vi "test Duplicate.vi"(8 "error in (no error)":errorcluster, 11 "TestCase In":refnum<class "Data Manipulation Tests.lvclass">) -> (0 "error out":errorcluster, 3 "TestCase Out":refnum<class "Data Manipulation Tests.lvclass">)   [LabVIEW 2017, in "Pointer Tests.lvlib" / "Data Manipulation Tests.lvclass"]
uses:
  Data Manipulation Tests.lvclass
  Source/Classes/Pointer/Public/New/New (4B).vi
  Source/Classes/Pointer/Public/Write/Write (1D I32).vi
  <vilib>/addons/_JKI Toolkits/VI Tester/TestCase.llb/TestCase.lvclass
  Source/Classes/Pointer/Pointer.lvclass
  C:/Program Files (x86)/National Instruments/LabVIEW 2017/vi.lib/addons/_JKI Toolkits/VI Tester/TestCase.llb/TestCase.lvclass
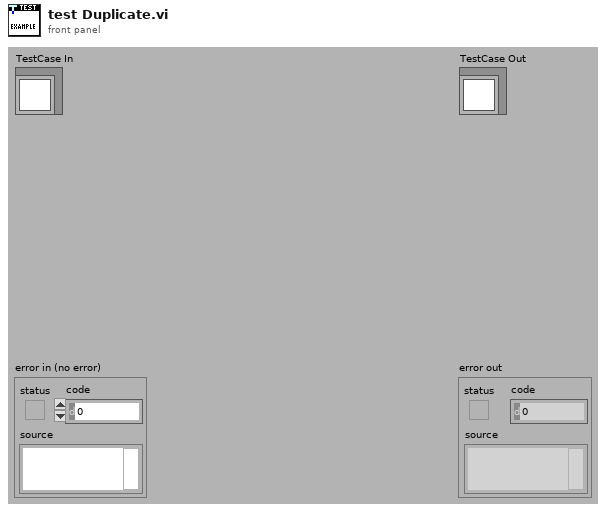
[diagram p1: front panel]
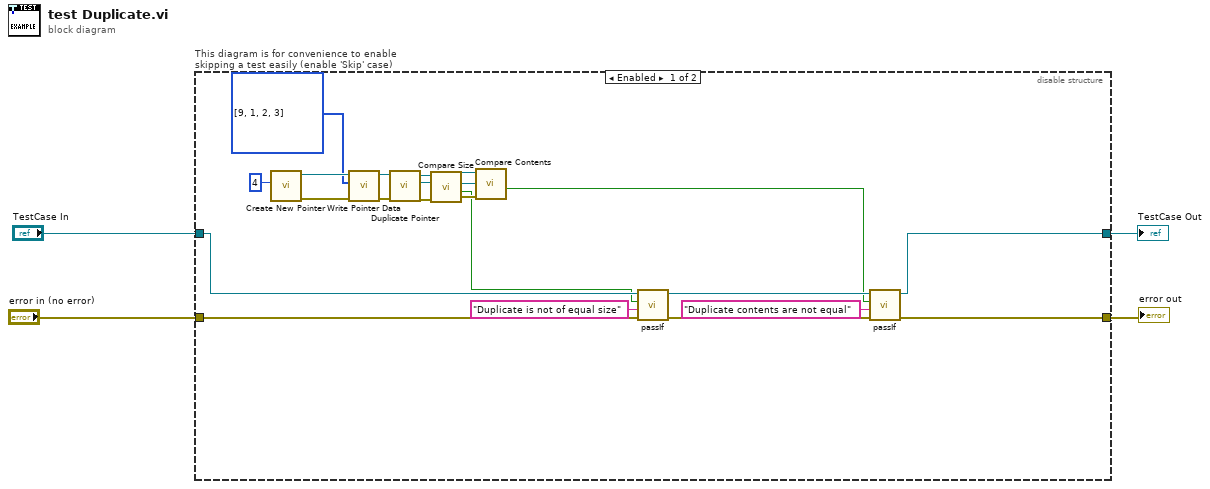
[diagram p0: block diagram]
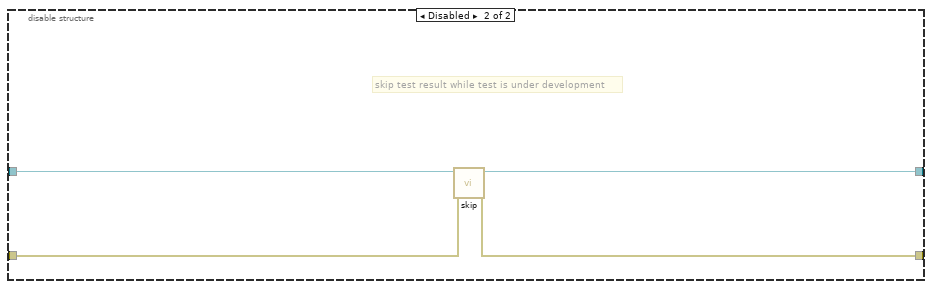
[diagram p2: hidden frame]
diagram:
  n1 = disable-structure "This diagram is for convenience to enable skipping a test easily (enable 'Skip' case)" shown="Enabled" {
    disable-tunnel: "TestCase In" -> [w23 w30]
    disable-tunnel: [w20 w28] -> w1
    disable-tunnel: [w22 w29] -> w3
    disable-tunnel: "error in (no error)" -> [w26 w27]
    frame Enabled {
      n2 = call-poly "Create New Pointer.vi"("count (1)"=u64 4) -> ("error out"=w8:errorcluster, "Pointer"=w25:refnum<class "Pointer.lvclass">)  [unwired: 9 in]
      n3 = call-poly "Write Pointer Data.vi"("error in (no error)"=w8, "buffer in"=i32[] [9, 1, 2, 3] ("count (1)"), "Pointer in"=w25) -> ("error out"=w7:errorcluster, "Pointer out"=w9:refnum<class "Pointer.lvclass">)  [unwired: 5 in, 2 out]
      n4 = call "Duplicate Pointer.vi"("error in (no error)"=w7, "Pointer in"=w9) -> ("error out"=w16:errorcluster, "new duplicate Pointer"=w13:refnum<class "Pointer.lvclass">, "Pointer out"=w17:refnum<class "Pointer.lvclass">)  [unwired: 7 in]
      n5 = call "Compare Size.vi"("error in (no error)"=w16, "Pointer b in"=w13, "Pointer a in"=w17) -> ("error out"=w14:errorcluster, "equal size?"=w11:bool, "Pointer b out"=w12:refnum<class "Pointer.lvclass">, "Pointer a out"=w15:refnum<class "Pointer.lvclass">)  [unwired: 5 in]
      n6 = call "Compare Contents.vi"("error in (no error)"=w14, "Pointer b in"=w12, "Pointer a in"=w15) -> ("equal contents?"=w10:bool)  [unwired: 5 in, 3 out]
      n7 = call-dynamic "passIf.vi"("error in (no error)"=w26, "message (\"\")"="Duplicate is not of equal size" ("message (\"\")"), "pass"=w11, "TestCase in"=w23) -> ("error out"=w24:errorcluster, "TestCase out"=w21:refnum<class "Data Manipulation Tests.lvclass">)  [unwired: 6 in]
      n8 = call-dynamic "passIf.vi"("error in (no error)"=w24, "message (\"\")"="Duplicate contents are not equal" ("message (\"\")"), "pass"=w10, "TestCase in"=w21) -> ("error out"=w22:errorcluster, "TestCase out"=w20:refnum<class "Data Manipulation Tests.lvclass">)  [unwired: 6 in]
    }
    frame Disabled {
      # "skip test result while test is under development"
      n9 = call <vilib>:"skip.vi"("error in (no error)"=w27, "TestCase in"=w30) -> ("error out"=w29:errorcluster, "TestCase out"=w28:refnum<class "Data Manipulation Tests.lvclass">)  [unwired: 8 in]
    }
  }
  "error out" <- w3
  "TestCase Out" <- w1
